vi "Randomize Tags.vi"(6 "error in (no error)":errorcluster, 8 "SwarmInputArray":T1(array[cluster]), 9 "TagArray In":refnum<class "Tag.lvclass">[](array[class]), 10 "Max H variatie":dbl, 11 "Max V variatie":dbl) -> (2 "New TagArray":refnum<class "Tag.lvclass">[](array[class]), 4 "error IO":errorcluster)   [LabVIEW 2014]
doc: "Generate and write new xy values for each Tag"
uses:
  Tag.lvclass
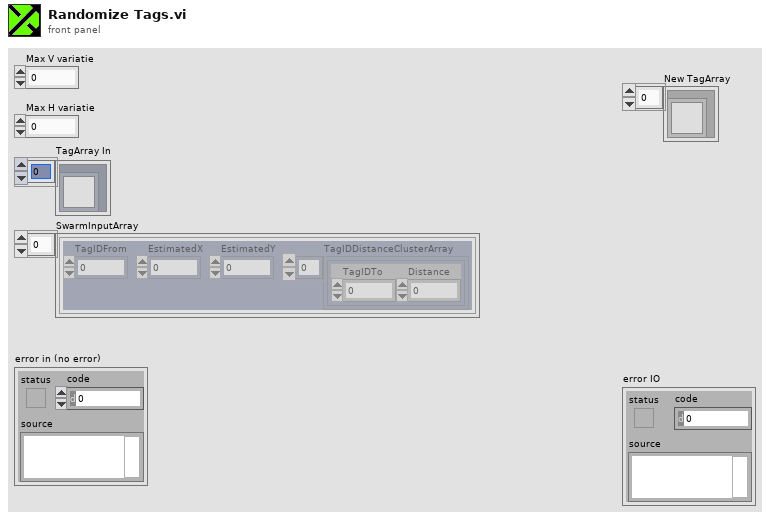
[diagram p1: front panel]
types:
  T1 = cluster{"TagIDFrom":dbl, "EstimatedX":dbl, "EstimatedY":dbl, "TagIDDistanceClusterArray":cluster{"TagIDTo":dbl, "Distance":dbl}[]}[]
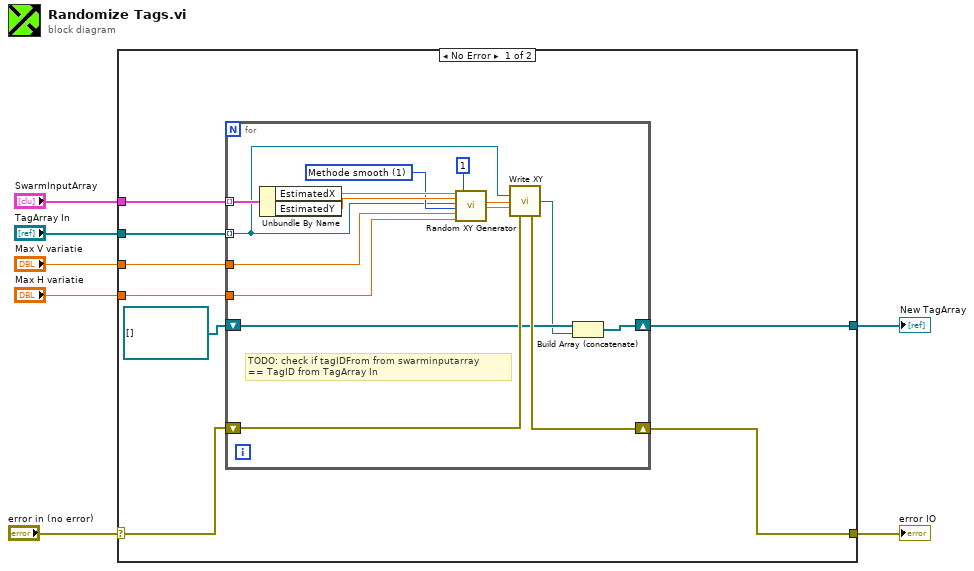
[diagram p0: block diagram]
diagram:
  n1 = case shown="No Error" "error in (no error)" {
    selector: "error in (no error)" -> [w11 w32]
    tunnel: [w10 w32] -> w6
    tunnel: "SwarmInputArray" -> [w15 _]
    tunnel: "TagArray In" -> [w14 w31]
    tunnel: "Max V variatie" -> [w13 _]
    tunnel: "Max H variatie" -> [w12 _]
    tunnel: [w9 w31] -> w1
    frame No Error {
      n2 = for {
        tunnel: w15 -> [w29] mode=indexing
        tunnel: w14 -> [w23] mode=indexing
        tunnel: w13 -> [w25]
        tunnel: w12 -> [w24]
        shift-right: [w21] -> w10
        shift-left: w11 -> [w22]
        shift-right: [w17] -> w9
        shift-left: refnum<class "Tag.lvclass">[] [] -> [w18]
        w26 = u16 1 items=["Methode Random", "Methode smooth"] ("Random Methode")
        # "TODO: check if tagIDFrom from swarminputarray\n== TagID from TagArray In"
        n3 = Unbundle By Name(w29) -> ("EstimatedX"=w28:dbl, "EstimatedY"=w27:dbl)
        n4 = call "Random XY Generator.vi"("X start"=w28, "Y start"=w27, "Tag.lvclass"=w23, "Random Methode"=w26, "MaxVelocity"=w25, "MaxHeading"=w24, "number of rounds"=1) -> ("x"=w20:dbl, "y"=w19:dbl)  [unwired: 9 in, 2 out]
        n5 = call "Write XY.vi"("Tag.lvclass"=w23, "TagX"=w20, "TagY"=w19, "error in (no error)"=w22) -> ("Tag Out"=w16:refnum<class "Tag.lvclass">, "error out"=w21:errorcluster)  [unwired: 10 in]
        n6 = Build Array (concatenate)(w18, w16) -> (w17:refnum<class "Tag.lvclass">[])
      }
    }
    frame Error {
    }
  }
  "error IO" <- w6
  "New TagArray" <- w1
